vi "format fpga settings.vi"(6 "scope settings":T5, 9 "Lockin":cluster{"LP BW (kHz)":dbl, "notch BW (kHz)":dbl}, 10 "PLL RF mixer":T3, 11 "PLL diode":T2) -> (1 "param PLL2":T1, 2 "param PLL2 2":T1, 3 "Cluster":cluster{dbl, dbl, dbl}, 4 "param Lockin":T4)   [LabVIEW 2018]
uses:
  scope settings.ctl
  PLL param interface.ctl
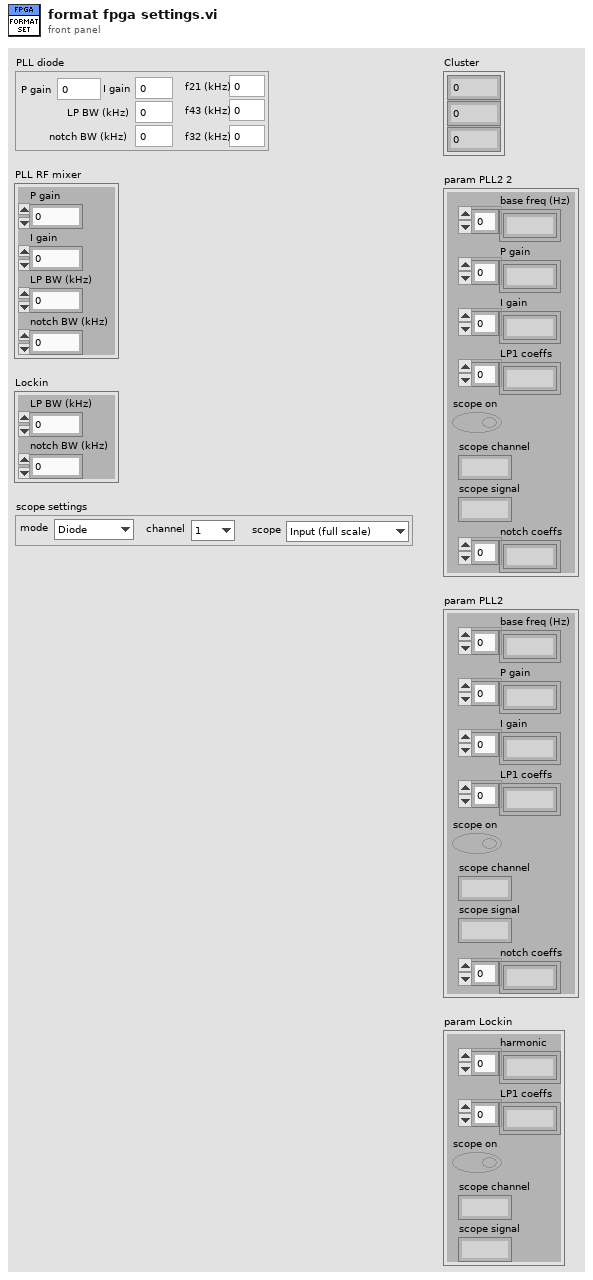
[diagram p1: front panel]
types:
  T1 = cluster{"base freq (Hz)":fxp<+,17,17>[], "P gain":fxp<+,14,14>[], "I gain":fxp<+,20,6>[], "LP1 coeffs":i32[], "scope on":bool, "scope channel":u8, "scope signal":u8, "notch coeffs":i32[]}
  T2 = typedef "PLL param interface.ctl" = cluster{"f21 (kHz)":dbl, "f43 (kHz)":dbl, "f32 (kHz)":dbl, "P gain":dbl, "I gain":dbl, "LP BW (kHz)":dbl, "notch BW (kHz)":dbl}
  T3 = cluster{"P gain":dbl, "I gain":dbl, "LP BW (kHz)":dbl, "notch BW (kHz)":dbl}
  T4 = cluster{"harmonic":fxp<+,20,6>[], "LP1 coeffs":i32[], "scope on":bool, "scope channel":u8, "scope signal":u8}
  T5 = typedef "scope settings.ctl" = cluster{"mode":enum16{"Diode", "RF mixer", "lockin"}, "channel":enum16{"1", "2", "3"}, "scope":enum16{"Input (full scale)", "PLL out", "Phase error (deg)", "Freq. error (Hz)"}}
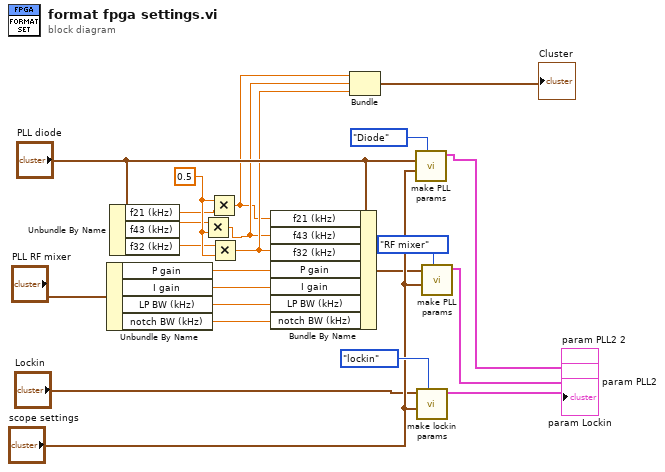
[diagram p0: block diagram]
diagram:
  w14 = 0.5 ("x")
  n1 = Unbundle By Name("PLL RF mixer") -> ("P gain"=w1:dbl, "I gain"=w2:dbl, "LP BW (kHz)"=w3:dbl, "notch BW (kHz)"=w4:dbl)
  n2 = Unbundle By Name("PLL diode") -> ("f21 (kHz)"=w5:dbl, "f43 (kHz)"=w6:dbl, "f32 (kHz)"=w7:dbl)
  n3 = Multiply(x=w6, y=w14) -> (x*y=w9:dbl)
  n4 = Multiply(x=w14, y=w5) -> (x*y=w8:dbl)
  n5 = Multiply(x=w7, y=w14) -> (x*y=w10:dbl)
  n6 = Bundle By Name(cluster="PLL diode", "f21 (kHz)"=w8, "f43 (kHz)"=w9, "f32 (kHz)"=w10, "P gain"=w1, "I gain"=w2, "LP BW (kHz)"=w3, "notch BW (kHz)"=w4) -> (w12:T2)
  n7 = Bundle(w8, w9, w10) -> (→"Cluster":cluster{dbl, dbl, dbl})  [unwired: 1 in]
  n8 = call "make PLL params.vi"("self"=enum16{"Diode", "RF mixer", "lockin"}."Diode", "scope settings"="scope settings", "PLL params in"="PLL diode") -> ("param PLL2"=→"param PLL2 2":T1)  [unwired: 8 in]
  n9 = call "make lockin params.vi"("self"=enum16{"Diode", "RF mixer", "lockin"}."lockin", "scope settings"="scope settings", "Lockin"="Lockin") -> ("param Lockin"=→"param Lockin":T4)  [unwired: 8 in]
  n10 = call "make PLL params.vi"("self"=enum16{"Diode", "RF mixer", "lockin"}."RF mixer", "scope settings"="scope settings", "PLL params in"=w12) -> ("param PLL2"=→"param PLL2":T1)  [unwired: 8 in]
